vi "Optical Lobe.vi"() -> ()   [LabVIEW 2011]
uses:
  WhereAmI.ctl
  <vilib>/userdefined/High Color/IMAQdx.ctl
  <vilib>/vision/Image Controls.llb/IMAQ Image.ctl
  OccGrid.ctl
  Position.ctl
  <vilib>/vision/driver/NI_Vision_Acquisition_Software.lvlib
panel:
  out "Image":T1(plugin-control)
  out "x":sgl[](array[numeric])
  out "y":sgl[](array[numeric])
  out "OccupancyGrid":i8[][](array[numeric])
  out "Working":bool
  in  "Camera/File?":bool
  in  "Camera Name":T2
  in  "Image file name":string="real pool targets rotated.bmp"
  out "Buoy 2":cluster{"x":sgl, "y":sgl}
  out "Bouy 1":cluster{"x":sgl, "y":sgl}
  out "Boat":T3
  out "Dock":cluster{"x":sgl, "y":sgl}
  in  "stop":bool
  out "error out":errorcluster
  out "Working Image":T1(plugin-control)
  # "File"
  # "Camera"
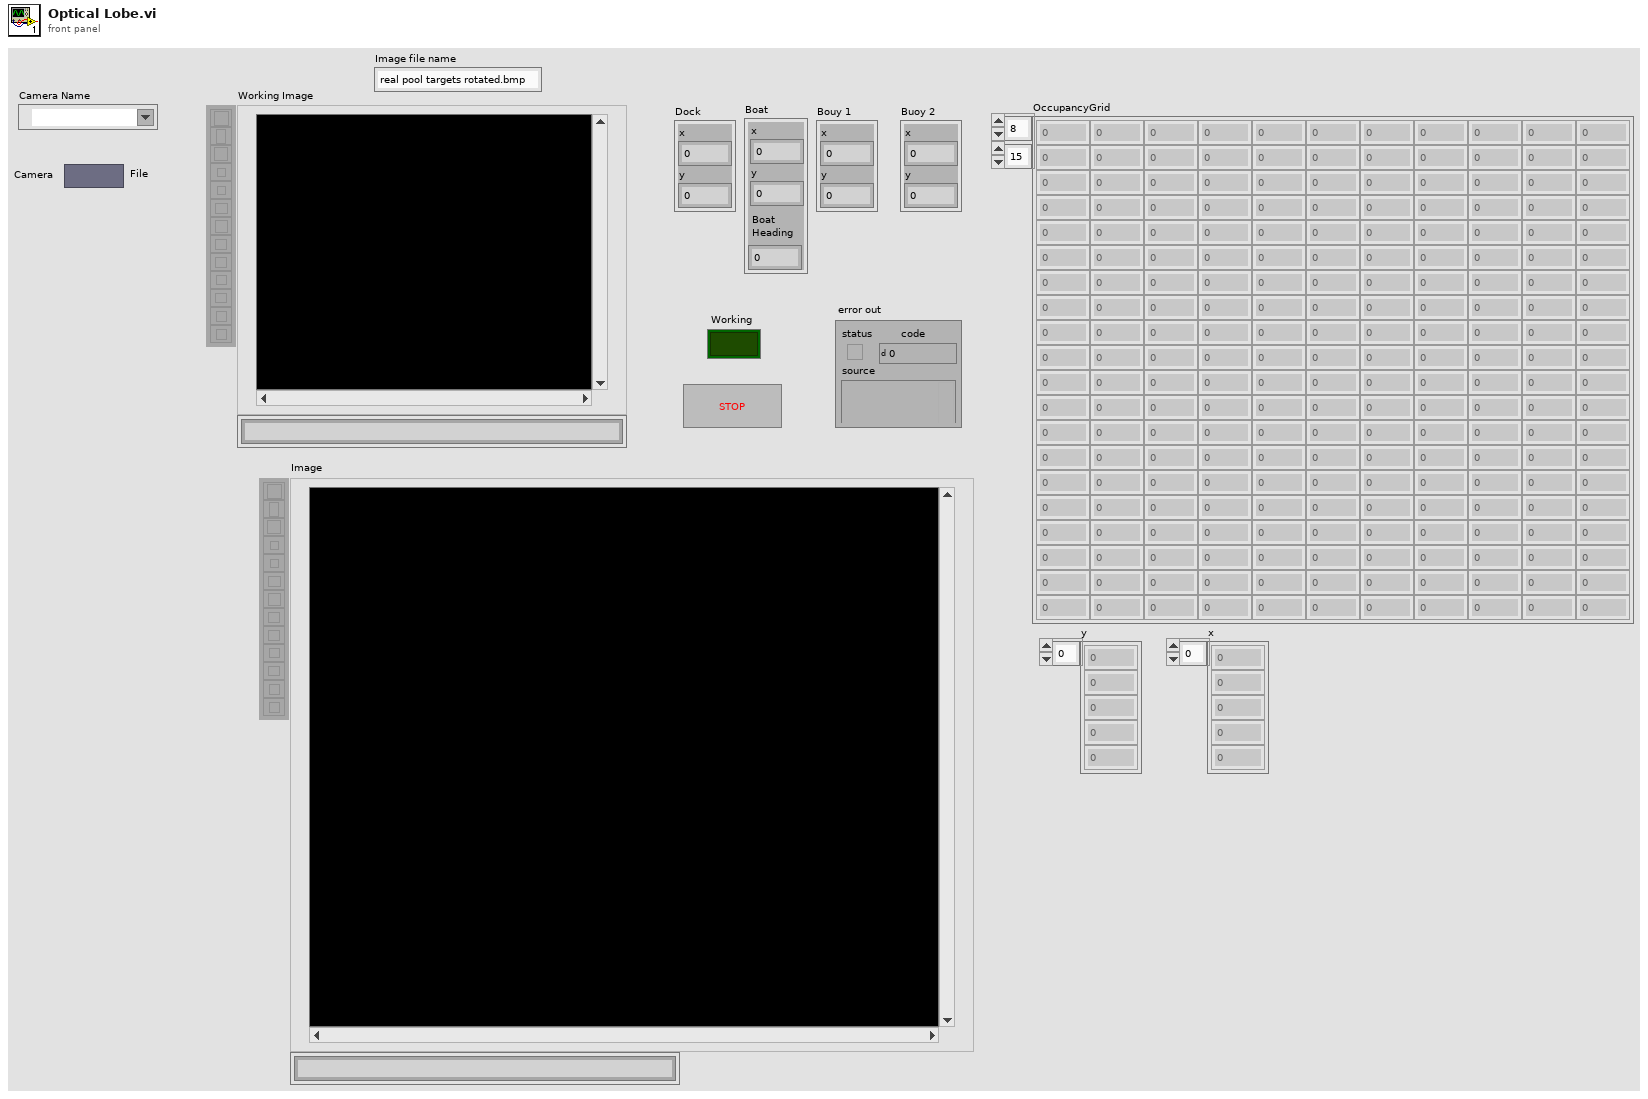
[diagram p1: front panel]
types:
  T1 = typedef "IMAQ Image.ctl" = refnum<image>
  T2 = typedef "IMAQdx.ctl" = refnum<k21>
  T3 = typedef "WhereAmI.ctl" = cluster{"x":sgl, "y":sgl, "Boat\nHeading":sgl}
  T4 = typedef "Image Type" = u32
  T5 = typedef "IMAQ GM Match Report.ctl" = cluster{"Position":cluster{"x":sgl, "y":sgl}, "Angle":sgl, "Scale":sgl, "Score":sgl, "Bounding Box":cluster{"x":sgl, "y":sgl}[], "Contrast Reversed":bool, "Occlusion %":sgl, "Template Target Curve Score":sgl, "Target Template Curve Score":sgl, "Correlation Score":sgl}
  T6 = cluster{"Position":cluster{"x":sgl, "y":sgl}, "Angle":sgl, "Scale":sgl, "Score":sgl, "Bounding Box":cluster{"x":sgl, "y":sgl}[]}[]
  T7 = cluster{"Position":cluster{"x":sgl, "y":sgl}, "Angle":sgl, "Scale":sgl, "Score":sgl, "Bounding Box":cluster{"x":sgl, "y":sgl}[]}
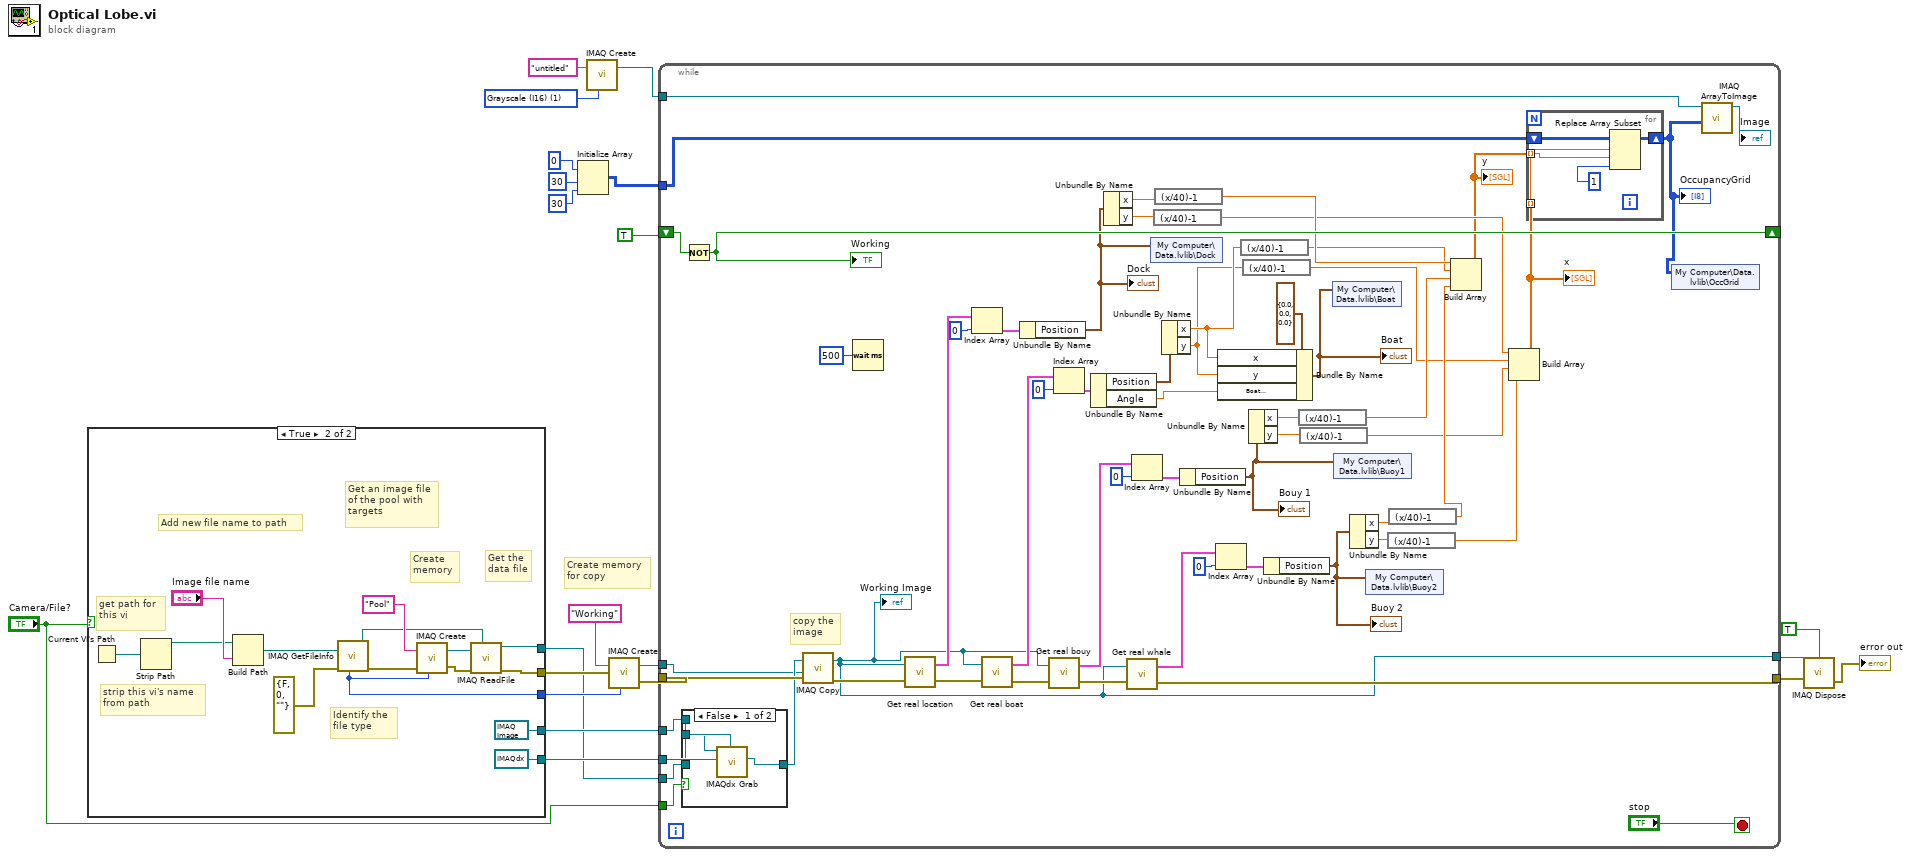
[diagram p0: block diagram]
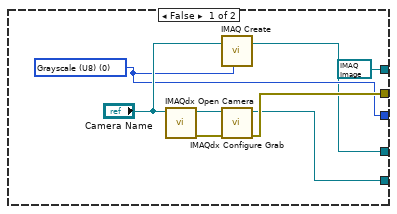
[diagram p3: hidden frame]
diagram:
  w4 = T4 1 items=["Grayscale (U8)", "Grayscale (I16)", "Grayscale (SGL)", "Complex (CSG)", "RGB (U32)", "HSL (U32)", "RGB (U64)", "Grayscale (U16)"] ("Image Type")
  # "Create memory\nfor copy"
  n1 = case shown="True" "Camera/File?" {
    tunnel: [T1 refnum ("Image Out") w34] -> w12
    tunnel: [w26 w33] -> w18
    tunnel: [w25 w32] -> w17
    tunnel: [w24 T1 refnum ("New Image")] -> w14
    tunnel: [w23 T2 refnum ("Session Out")] -> w13
    frame False {
      w25 = T4 0 items=["Grayscale (U8)", "Grayscale (I16)", "Grayscale (SGL)", "Complex (CSG)", "RGB (U32)", "HSL (U32)", "RGB (U64)", "Grayscale (U16)"] ("Image Type")
      n2 = call <vilib>:"IMAQdx Open Camera.vi"("Session In"="Camera Name") -> ("error out"=w29:errorcluster, "Session Out"=w28:T2)  [unwired: 2 in, 7 out]
      n3 = call "IMAQ Create"("Image Name"="Camera Name", "Image Type"=w25) -> ("New Image"=w24:T1)  [unwired: 2 in, 2 out]
      n4 = call <vilib>:"IMAQdx Configure Grab.vi"("error in"=w29, "Session In"=w28) -> ("error out"=w26:errorcluster, "Session Out"=w23:T2)  [unwired: 8 out]
    }
    frame True {
      # "Add new file name to path"
      # "strip this vi's name \nfrom path"
      # "get path for \nthis vi"
      # "Get the \ndata file"
      # "Create \nmemory"
      # "Identify the \nfile type"
      # "Get an image file\nof the pool with\ntargets"
      n5 = Current VI's Path() -> (path=w37:path)
      n6 = Strip Path(path=w37) -> (stripped path=w36:path)  [unwired: 1 out]
      n7 = Build Path(base path=w36, name or relative path="Image file name") -> (appended path=w35:path)
      n8 = call "IMAQ GetFileInfo"("error in (no error)"=errorcluster {"status"=FALSE, "code"=0, "source"=""}, "File Path"=w35) -> ("error out"=w43:errorcluster, "Image Type"=w32:T4)  [unwired: 3 in, 5 out]
      n9 = call "IMAQ Create"("Image Name"="Pool", "Image Type"=w32, "error in (no error)"=w43) -> ("New Image"=w41:T1, "error out"=w39:errorcluster)  [unwired: 2 in]
      n10 = call "IMAQ ReadFile"("File Path"=w35, "error in (no error)"=w39, "Image"=w41) -> ("error out"=w33:errorcluster, "Image Out"=w34:T1)  [unwired: 4 in, 3 out]
    }
  }
  n11 = Initialize Array(i16 0 ("element"), 30 ("dimension size"), 30 ("dimension size")) -> (w6:i16[][])
  n12 = call "IMAQ Create"("Image Name"="untitled", "Image Type"=w4) -> ("New Image"=w5:T1)  [unwired: 3 in, 1 out]
  n13 = call "IMAQ Create"("Image Name"="Working", "Image Type"=w17, "error in (no error)"=w18) -> ("New Image"=w19:T1, "error out"=w21:errorcluster)  [unwired: 2 in]
  n14 = while {
    tunnel: w21 -> [w101]
    tunnel: w19 -> [w69]
    tunnel: [w84] -> w2
    tunnel: [w83] -> w16
    tunnel: w14 -> [w80]
    tunnel: w13 -> [w79]
    tunnel: w12 -> [w78]
    tunnel: "Camera/File?" -> [w76]
    shift-right: [w74] -> _
    shift-left: TRUE -> [w75]
    tunnel: w6 -> [w65]
    tunnel: w5 -> [w45]
    stop <- "stop" stop-if-true
    # "copy the\nimage"
    n15 = case shown="False" w76 {
      tunnel: w80 -> [w109 _]
      tunnel: w79 -> [w108 _]
      tunnel: w78 -> [_ w110]
      tunnel: [w107 w110] -> w77
      frame False {
        n16 = call <vilib>:"IMAQdx Grab.vi"("Image In"=w109, "Session In"=w108) -> ("Image Out"=w107:T1)  [unwired: 2 in, 7 out]
      }
      frame True {
      }
    }
    n17 = Not(x=w75) -> (.not. x?=w74:bool)
    "Working" <- w74
    n18 = call "IMAQ Copy"("error in (no error)"=w101, "Image Dst"=w69, "Image Src"=w77) -> ("error out"=w86:errorcluster, "Image Dst Out"=w83:T1)  [unwired: 3 in]
    "Working Image" <- w83
    n19 = Wait (ms)(milliseconds to wait=u32 500) -> ()  [unwired: 1 out]
    n20 = call "Get real location.vi"("error in"=w86, "Image"=w83) -> ("error out"=w98:errorcluster, "Matches"=w99:T5[])
    n21 = Index Array(array=w99, index=0) -> (element=w100:T5)
    n22 = call "Get real boat.vi"("error in"=w98, "Image"=w83) -> ("error out"=w93:errorcluster, "Matches"=w94:T5[])
    n23 = Unbundle By Name(w100) -> ("Position"=w68:cluster{"x":sgl, "y":sgl})
    "Dock" <- w68
    n24 = call "Get real bouy.vi"("error in"=w93, "Image"=w83) -> ("error out"=w89:errorcluster, "Matches"=w90:T5[])
    n25 = Index Array(array=w94, index=0) -> (element=w96:T5)
    n26 = Unbundle By Name(w96) -> ("Position"=w73:cluster{"x":sgl, "y":sgl}, "Angle"=w72:sgl)
    n27 = Unbundle By Name(w68) -> ("x"=w67:sgl, "y"=w66:sgl)
    n28 = call "Get real whale.vi"("error in"=w89, "Image"=w83) -> ("error out"=w84:errorcluster, "Matches"=w85:T6)
    n29 = Index Array(array=w90, index=0) -> (element=w91:T5)
    n30 = shared-variable "My Computer\\Data.lvlib\\Dock"(w68) -> ()  [unwired: 1 in, 1 out]
    n31 = expression code="(x/40)-1"(w66) -> (w52:sgl)
    n32 = expression code="(x/40)-1"(w67) -> (w56:sgl)
    n33 = Unbundle By Name(w73) -> ("x"=w64:sgl, "y"=w63:sgl)
    n34 = Unbundle By Name(w91) -> ("Position"=w62:cluster{"x":sgl, "y":sgl})
    "Bouy 1" <- w62
    n35 = Index Array(array=w85, index=0) -> (element=w88:T7)
    n36 = Bundle By Name(cluster=T3 {"x"=0.0, "y"=0.0, "Boat\nHeading"=0.0} ("Boat"), "x"=w64, "y"=w63, "Boat\nHeading"=w72) -> (w70:T3)
    "Boat" <- w70
    n37 = expression code="(x/40)-1"(w64) -> (w55:sgl)
    n38 = expression code="(x/40)-1"(w63) -> (w51:sgl)
    n39 = Unbundle By Name(w62) -> ("x"=w61:sgl, "y"=w60:sgl)
    n40 = Unbundle By Name(w88) -> ("Position"=w59:cluster{"x":sgl, "y":sgl})
    "Buoy 2" <- w59
    n41 = expression code="(x/40)-1"(w61) -> (w54:sgl)
    n42 = expression code="(x/40)-1"(w60) -> (w50:sgl)
    n43 = shared-variable "My Computer\\Data.lvlib\\Boat"(w70) -> ()  [unwired: 1 in, 1 out]
    n44 = shared-variable "My Computer\\Data.lvlib\\Buoy1"(w62) -> ()  [unwired: 1 in, 1 out]
    n45 = Unbundle By Name(w59) -> ("x"=w58:sgl, "y"=w57:sgl)
    n46 = shared-variable "My Computer\\Data.lvlib\\Buoy2"(w59) -> ()  [unwired: 1 in, 1 out]
    n47 = expression code="(x/40)-1"(w57) -> (w49:sgl)
    n48 = expression code="(x/40)-1"(w58) -> (w53:sgl)
    n49 = Build Array(w56, w55, w54, w53) -> (w48:sgl[])
    "y" <- w48
    n50 = Build Array(w52, w51, w50, w49) -> (w47:sgl[])
    "x" <- w47
    n51 = for {
      tunnel: w48 -> [w105] mode=indexing
      tunnel: w47 -> [w104] mode=indexing
      shift-right: [w102] -> w44
      shift-left: w65 -> [w106]
      n52 = Replace Array Subset(array=w106, new element=i8 1 ("new element/subarray"), index (row)=w104, index (col)=w105) -> (w102:i16[][])
    }
    "OccupancyGrid" <- w44
    n53 = shared-variable "My Computer\\Data.lvlib\\OccGrid"(w44) -> ()  [unwired: 1 in, 1 out]
    n54 = call "IMAQ ArrayToImage"("Image Pixels (I16)"=w44, "Image"=w45) -> ("Image Out"=→"Image":T1)  [unwired: 8 in, 1 out]
  }
  n55 = call "IMAQ Dispose"("All Images? (No)"=TRUE, "Image"=w16, "error in (no error)"=w2) -> ("error out"=→"error out":errorcluster)  [unwired: 3 in]
